vi "GetText.vi"(8 "error in":errorcluster, 11 "node in":refnum<class "Target.lvclass">) -> (0 "error out":errorcluster, 1 "additional text":string, 2 "text":string, 3 "node out":refnum<class "Target.lvclass">, 4 "glyph":string)   [LabVIEW 2015, in "Target.lvclass"]
doc: "Returns the text representation of the node used for the tree control."
uses:
  Target.lvclass
  Target.lvclass/Target.ctl
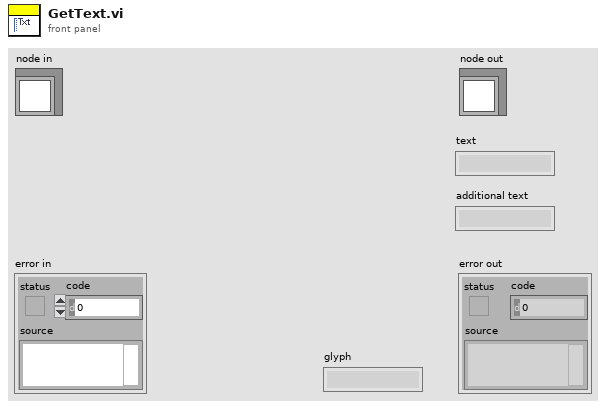
[diagram p1: front panel]
types:
  T1 = typedef "VeriStand XML Parser.lvlib/Supported Targets.ctl" = enum16{"All", "Pharlap", "VxWorks", "Windows", "Linux_32_ARM", "Linux_x64", "PharlapWindows", "PharlapVxWorks", "VxWorksWindows"}
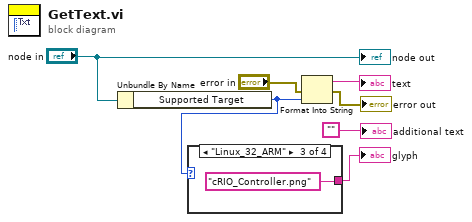
[diagram p0: block diagram]
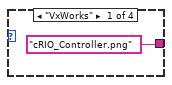
[diagram p2: hidden frame]
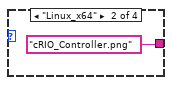
[diagram p3: hidden frame]
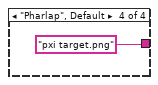
[diagram p4: hidden frame]
diagram:
  n1 = Unbundle By Name("node in") -> ("Supported Target"=w2:T1)
  n2 = case shown="\"Linux_32_ARM\"" w2 {
    tunnel: ["cRIO_Controller.png" ("glyph") "cRIO_Controller.png" ("glyph") "cRIO_Controller.png" ("glyph") "pxi target.png" ("glyph")] -> w1
    frame "VxWorks" {
    }
    frame "Linux_x64" {
    }
    frame "Linux_32_ARM" {
    }
    frame "Pharlap", Default {
    }
  }
  "glyph" <- w1
  n3 = Format Into String(error in="error in", w2) -> (resulting string=→"text":string, error out=→"error out":errorcluster)  [unwired: 2 in]
  "node out" <- "node in"
  "additional text" <- ""
